vi "Certaintygraph test.vi"() -> ()   [LabVIEW 2012]
uses:
  <vilib>/FPGAPlugInAG/sbRIO-9636/niLvFpga_Open_sbRIO-9636.vi
  <vilib>/rvi/interface/common/dynamic/niFpgaDynamicAddResources.vi
  <vilib>/Utility/error.llb/Error Cluster From Error Code.vi
  <vilib>/rvi/errors/niLvFpgaAdjustHostInterfaceError.vi
  <vilib>/FPGAPlugInAG/Dynamic/niLvFpga_Close_Dynamic.vi
  <vilib>/rvi/interface/nirviOpenFPGA/nirviOpenFPGA.xnode
  FPGA Bitfiles/NIARCDemo-kyle_FPGATarget_FPGAToplevel_9c4As6+H2cU.lvbitx
  <vilib>/rvi/interface/nirviReadWriteControl/nirviReadWriteControl.xnode
  <vilib>/rvi/interface/nirviCloseFPGA/nirviCloseFPGA.xnode
  NiFpgaLv.dll
  <vilib>/rvi/interface/Simulation/niFpgaSimulationCallBeginRW.vi
panel:
  out "distance left":fxp<+/-,64,32>
  out "distance right":fxp<+/-,64,32>
  in  "Sensor y":i16
  in  "Sensor x":i16
  in  "stop":bool
  out "distance front":fxp<+/-,64,32>
  in  "Degrees":dbl
  out "Intensity Graph":i16[][](graph)
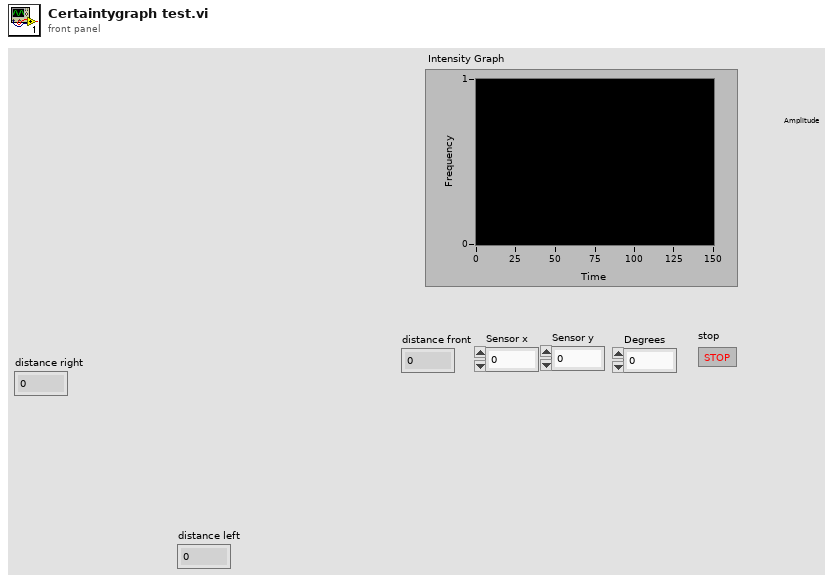
[diagram p1: front panel]
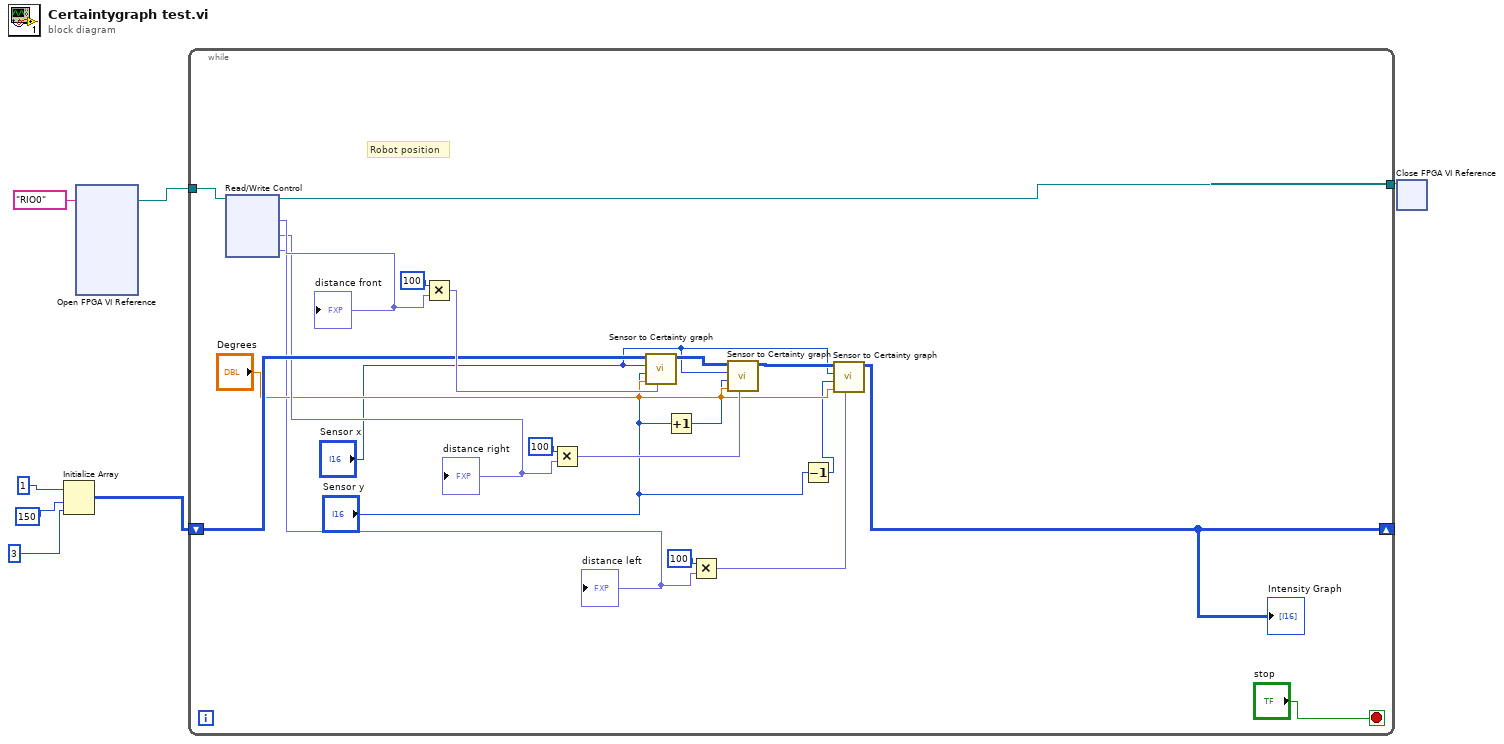
[diagram p0: block diagram]
diagram:
  n1 = Initialize Array(i16 1, i16 150, 3) -> (w3:i16[][])
  n2 = xnode "Open FPGA VI Reference"("resource name"=tag "RIO0") -> ("FPGA VI Reference Out"=w7:refnum<k20>)  [unwired: 1 in, 1 out]
  n3 = while {
    tunnel: w7 -> [w28]
    tunnel: [w27] -> w6
    shift-right: [w8] -> _
    shift-left: w3 -> [w22]
    stop <- "stop" stop-if-true
    # "Robot position"
    n4 = xnode "Read/Write Control"("FPGA VI Reference In"=w28) -> ("FPGA VI Reference Out"=w27:refnum<k20>, "IR 0"=w24:fxp<+/-,24,5>, "IR 1"=w20:fxp<+/-,24,5>, "IR 2"=w10:fxp<+/-,24,5>)  [unwired: 1 in, 1 out]
    "distance front" <- w24
    "distance right" <- w20
    "distance left" <- w10
    n5 = Multiply(x=100, y=w24) -> (x*y=w23:fxp<+/-,56,37>)
    n6 = Multiply(x=100, y=w20) -> (x*y=w19:fxp<+/-,56,37>)
    n7 = call "Sensor to Certainty graph.vi"("Distance"=w23, "Degrees"="Degrees", "Sensor y"="Sensor y", "Sensor x"="Sensor x", "Array 2"=w22) -> ("Array 3"=w18:i16[][])  [unwired: 6 in]
    n8 = Increment(x="Sensor y") -> (x+1=w15:i16)
    n9 = Multiply(x=100, y=w10) -> (x*y=w9:fxp<+/-,56,37>)
    n10 = call "Sensor to Certainty graph.vi"("Distance"=w19, "Degrees"="Degrees", "Sensor y"=w15, "Sensor x"="Sensor x", "Array 2"=w18) -> ("Array 3"=w17:i16[][])  [unwired: 6 in]
    n11 = Decrement(x="Sensor y") -> (x-1=w13:i16)
    n12 = call "Sensor to Certainty graph.vi"("Distance"=w9, "Degrees"="Degrees", "Sensor y"=w13, "Sensor x"="Sensor x", "Array 2"=w17) -> ("Array 3"=w8:i16[][])  [unwired: 6 in]
    "Intensity Graph" <- w8
  }
  n13 = xnode "Close FPGA VI Reference"("FPGA VI Reference In"=w6) -> ()  [unwired: 1 in, 1 out]
